vi "MiniCompareDelete.vi"(6 "Value":i32, 8 "output array 2":dbl[][](array[numeric]), 10 "Veri Aralığı":i32[](array[numeric])) -> (2 "output array 3":dbl[][](array[numeric]), 3 "CompareXY 2":T1(graph))   [LabVIEW 2021]
panel:
  in  "Alt Limit":string
  out "Numeric 4":i32
  out "Numeric 3":i32
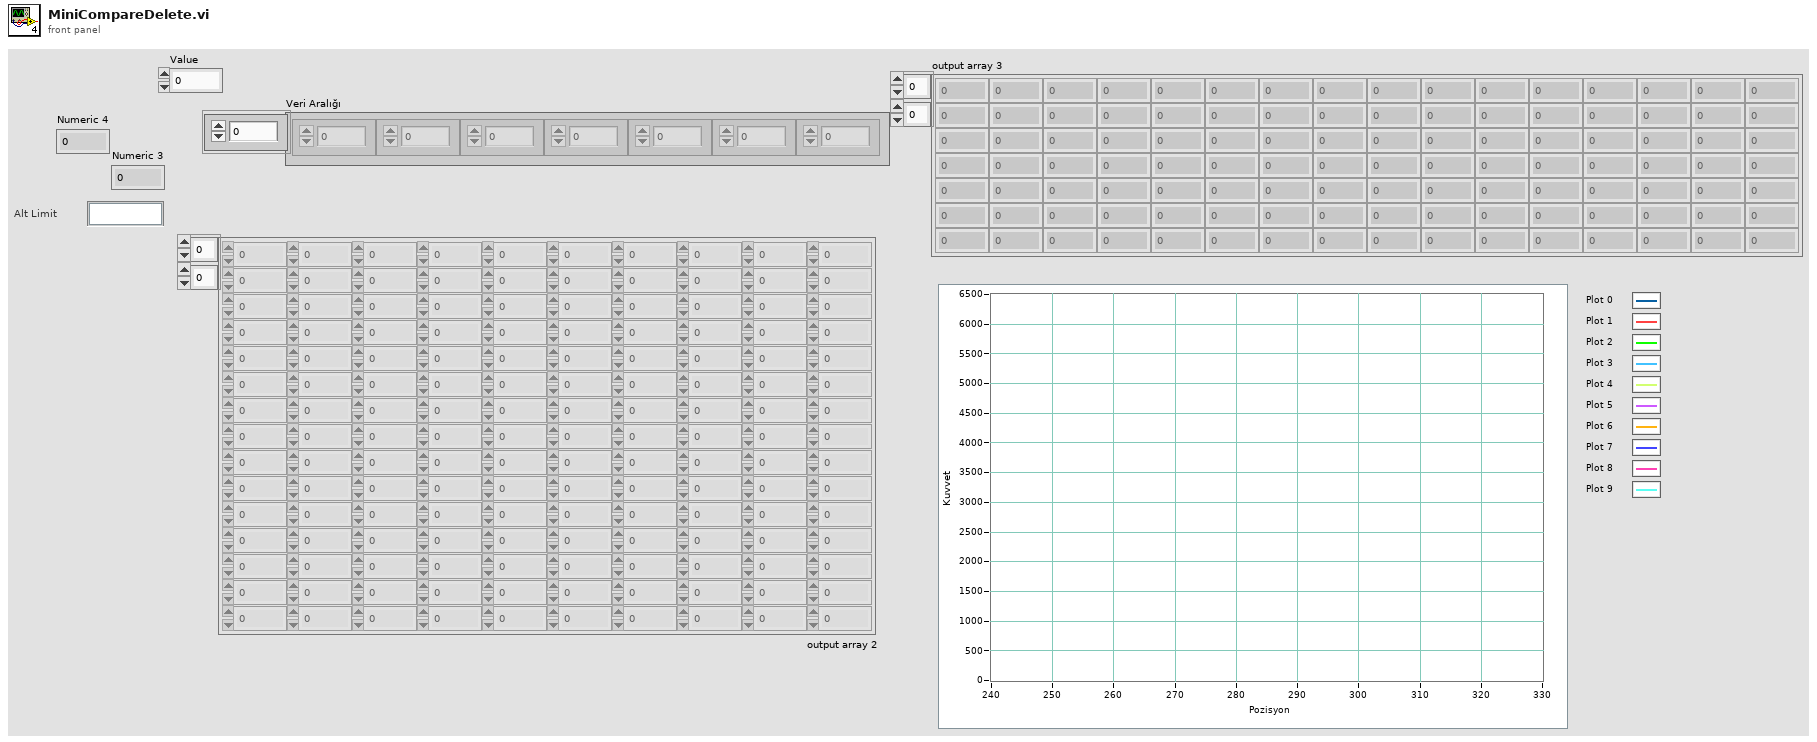
[diagram p1: front panel]
types:
  T1 = cluster{"Item Names":dbl[], "Item Names":dbl[]}[]
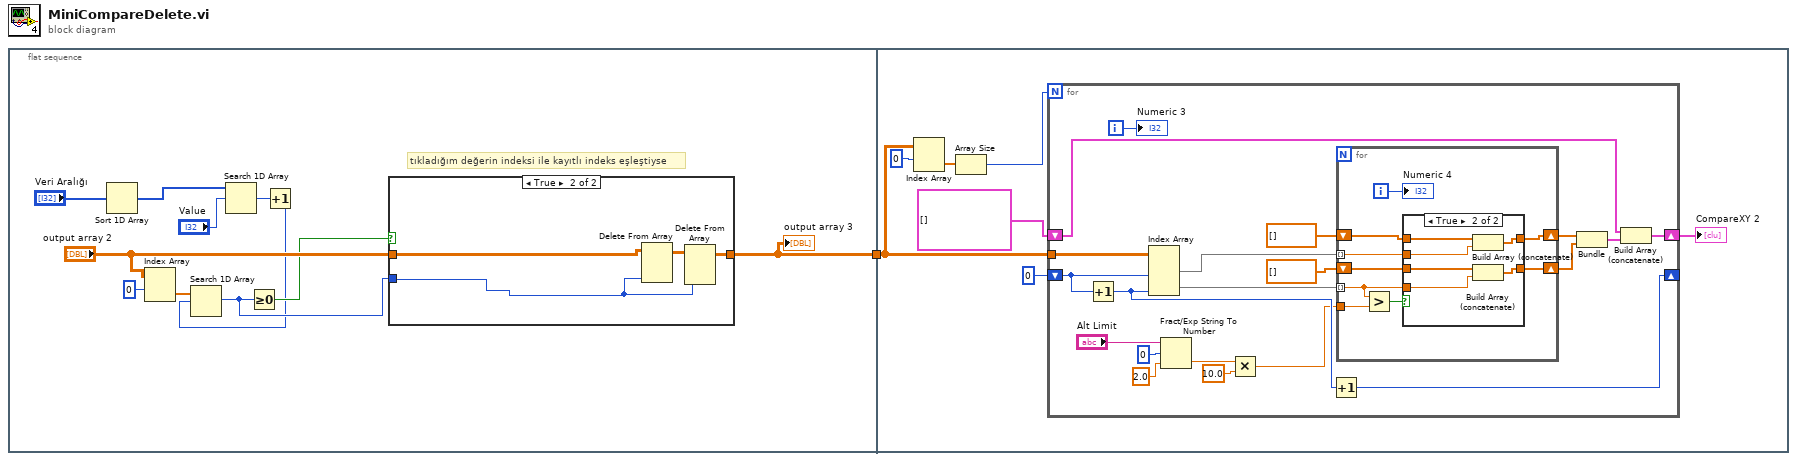
[diagram p0: block diagram]
diagram:
  n1 = flat-sequence {
    tunnel: [w12] -> w1
    tunnel: w1 -> [w18]
    frame #0 {
      # "tıkladığım değerin indeksi ile kayıtlı indeks eşleştiyse"
      n2 = Sort 1D Array(array="Veri Aralığı") -> (sorted array=w4:i32[])
      n3 = Index Array(array="output array 2", index (row)=0) -> (element=w7:dbl[])  [unwired: 1 in]
      n4 = Search 1D Array(1D array=w4, element="Value") -> (index of element=w3:i32)  [unwired: 1 in]
      n5 = Increment(x=w3) -> (x+1=w2:i32)
      n6 = Search 1D Array(1D array=w7, element=w2) -> (index of element=w5:i32)  [unwired: 1 in]
      n7 = Greater Or Equal To 0?(x=w5) -> (x >= 0?=w6:bool)
      n8 = case shown="True" w6 {
        tunnel: [w13 w15] -> w12
        tunnel: "output array 2" -> [w13 w16]
        tunnel: w5 -> [_ w14]
        frame False {
        }
        frame True {
          n9 = Delete From Array(array=w16, index (col)=w14) -> (array with subset deleted=w17:dbl[][])  [unwired: 2 in, 1 out]
          n10 = Delete From Array(array=w17, index (col)=w14) -> (array with subset deleted=w15:dbl[][])  [unwired: 2 in, 1 out]
        }
      }
      "output array 3" <- w12
    }
    frame #1 {
      n11 = Index Array(array=w18, index (row)=0) -> (element=w24:dbl[])  [unwired: 1 in]
      n12 = Array Size(array=w24) -> (size(s)=w23:i32)
      n13 = for {
        N: w23 -> [_]
        tunnel: w18 -> [w25]
        shift-right: [w43] -> _
        shift-left: 0 -> [w44]
        shift-right: [w39] -> w22
        shift-left: T1 [] -> [w40]
        i -> [w30]
        n14 = Increment(x=w44) -> (x+1=w42:i32)
        n15 = Index Array(array=w25, index (col) #1=w44, index (col) #2=w42) -> (element #1=w35:dbl[], element #2=w36:dbl[])  [unwired: 2 in]
        n16 = Fract/Exp String To Number(string="Alt Limit", offset=0, default (0 dbl)=2.0 ("default (0 DBL)")) -> (number=w28:dbl)  [unwired: 1 in, 1 out]
        n17 = Multiply(x=w28, y=10.0) -> (x*y=w27:dbl)
        n18 = Increment(x=w42) -> (x+1=w43:i32)
        n19 = for {
          tunnel: w27 -> [w53]
          tunnel: w36 -> [w45] mode=indexing
          shift-right: [w51] -> w33
          shift-left: dbl[] [] -> [w52]
          tunnel: w35 -> [w46] mode=indexing
          shift-right: [w47] -> w34
          shift-left: dbl[] [] -> [w50]
          i -> [w49]
          n20 = Greater?(x=w45, y=w53) -> (0:w48:bool)
          n21 = case shown="True" w48 {
            tunnel: w52 -> [w55 w61]
            tunnel: [w55 w60] -> w51
            tunnel: w45 -> [_ w56]
            tunnel: w46 -> [_ w57]
            tunnel: w50 -> [w54 w59]
            tunnel: [w54 w58] -> w47
            frame False {
            }
            frame True {
              n22 = Build Array (concatenate)(w59, w57) -> (w58:dbl[])
              n23 = Build Array (concatenate)(w61, w56) -> (w60:dbl[])
            }
          }
          "Numeric 4" <- w49
        }
        n24 = Bundle(w34, w33) -> (w41:cluster{dbl[], dbl[]})  [unwired: 1 in]
        n25 = Build Array (concatenate)(w40, w41) -> (w39:T1)
        "Numeric 3" <- w30
      }
      "CompareXY 2" <- w22
    }
  }
